vi "nanocal -- nuclear schottky goodness V4.vi"(6 "parameters IN":map{T1, dbl}(c390), 7 "weighting strategy":T2, 8 "dz/dω IN (V)":cdb[](array[numeric])=[1.7183506006211996e-05+0.0i, 1.7124360968751133e-05+0.0i, 1.7049104347380084e-05+0.0i, 1.700437896335042e-05+0.0i, 1.6984579723285106e-05+0.0i, 1.702277369054923e-05+0.0i, 1.713094025845651e-05+0.0i, 1.734249707866828e-05+0.0i, 1.768320429215342e-05+0.0i, 1.8195281152538477e-05+0.0i, 1.8917228661806973e-05+0.0i, 1.9897834564883332e-05+0.0i, 2.154104046962704e-05+0.0i, 2.3247799321765792e-05+0.0i, 2.5364678450551808e-05+0.0i, 2.8645788781885885e-05+0.0i, 3.204749554800641e-05+0.0i, 3.783559691555022e-05+0.0i, 4.245015867332296e-05+0.0i, 4.909131821431355e-05+0.0i, 5.511821898441184e-05+0.0i, 6.178843506022867e-05+0.0i, 7.1079604965352e-05+0.0i, 7.922304381453334e-05+0.0i, 8.814778883893872e-05+0.0i, 9.806709148886077e-05+0.0i, 0.00011119043245647465+0.0i, 0.00012253184919712196+0.0i, 0.00013777724317049346+0.0i, 0.0001508081004573332+0.0i, 0.00016547294918783876+0.0i, 0.00018003847596605868+0.0i, 0.00019518361086534857+0.0i, 0.00021134179818259658+0.0i, 0.0002372041782935464+0.0i, 0.00025518143132024254+0.0i, 0.0002835129702467886+0.0i, 0.0003060118087631287+0.0i, 0.00032860772064336976+0.0i, 0.0003492674091322389+0.0i, 0.00037498324855458583+0.0i, 0.00040021078021115026+0.0i, 0.00041969942568205823+0.0i, 0.00044367338947118773+0.0i, 0.0004634793607238068+0.0i, 0.00047921028781215815+0.0i, 0.0004880906353641744+0.0i, 0.0004932212623741357+0.0i, 0.000491476456593048+0.0i, 0.000480893803992059+0.0i, 0.0004535995818650303+0.0i, 0.000417087772881063+0.0i, 0.0003564148692854789+0.0i, 0.0003049201646356487+0.0i, 0.00021260191240459413+0.0i, 0.00011714858948470126+0.0i, 1.675457544365132e-05+0.0i, -6.8674075405897e-05+0.0i, -0.000156473047607305+0.0i, -0.00026709373934749337+0.0i, -0.0003544271565676041+0.0i, -0.00047937600197311275+0.0i, -0.0006086290582260493+0.0i, -0.0007031877411848573+0.0i, -0.0007564526901441745+0.0i, -0.000802489180995596+0.0i, -0.0008414596018105983+0.0i, -0.0008809346482248761+0.0i, -0.0009073902840241921+0.0i, -0.0009264953054508651+0.0i, -0.0009405659412141811+0.0i, -0.000951649722530156+0.0i, -0.0009557485581057351+0.0i, -0.0009558464741053665+0.0i, -0.0009509110176922098+0.0i, -0.0009411315169847015+0.0i, -0.0009303400913929496+0.0i, -0.0009171113529290538+0.0i, -0.0009022111527275027+0.0i, -0.0008813746494947608+0.0i, -0.0008581837971946129+0.0i, -0.0008372063466683705+0.0i, -0.0008165626610594428+0.0i, -0.0007901155435838691+0.0i, -0.0007682834352800848+0.0i, -0.000746231015527196+0.0i, -0.0007238798463130141+0.0i, -0.0007015567569177018+0.0i, -0.000679301954671598+0.0i, -0.0006572001413831251+0.0i, -0.000629855254567978+0.0i, -0.0006083942229188815+0.0i, -0.0005768631156754208+0.0i, -0.0005562177438951648+0.0i, -0.0005359092039599222+0.0i, -0.0005145186443378148+0.0i, -0.0004951602053444319+0.0i, -0.00047624970229075174+0.0i, -0.0004577401041527736+0.0i, -0.00043519037796120065+0.0i], 9 "Voltage IN (V)":cdb[](array[numeric])=[1.7183506006211996e-05+0.0i, 1.7124360968751133e-05+0.0i, 1.7049104347380084e-05+0.0i, 1.700437896335042e-05+0.0i, 1.6984579723285106e-05+0.0i, 1.702277369054923e-05+0.0i, 1.713094025845651e-05+0.0i, 1.734249707866828e-05+0.0i, 1.768320429215342e-05+0.0i, 1.8195281152538477e-05+0.0i, 1.8917228661806973e-05+0.0i, 1.9897834564883332e-05+0.0i, 2.154104046962704e-05+0.0i, 2.3247799321765792e-05+0.0i, 2.5364678450551808e-05+0.0i, 2.8645788781885885e-05+0.0i, 3.204749554800641e-05+0.0i, 3.783559691555022e-05+0.0i, 4.245015867332296e-05+0.0i, 4.909131821431355e-05+0.0i, 5.511821898441184e-05+0.0i, 6.178843506022867e-05+0.0i, 7.1079604965352e-05+0.0i, 7.922304381453334e-05+0.0i, 8.814778883893872e-05+0.0i, 9.806709148886077e-05+0.0i, 0.00011119043245647465+0.0i, 0.00012253184919712196+0.0i, 0.00013777724317049346+0.0i, 0.0001508081004573332+0.0i, 0.00016547294918783876+0.0i, 0.00018003847596605868+0.0i, 0.00019518361086534857+0.0i, 0.00021134179818259658+0.0i, 0.0002372041782935464+0.0i, 0.00025518143132024254+0.0i, 0.0002835129702467886+0.0i, 0.0003060118087631287+0.0i, 0.00032860772064336976+0.0i, 0.0003492674091322389+0.0i, 0.00037498324855458583+0.0i, 0.00040021078021115026+0.0i, 0.00041969942568205823+0.0i, 0.00044367338947118773+0.0i, 0.0004634793607238068+0.0i, 0.00047921028781215815+0.0i, 0.0004880906353641744+0.0i, 0.0004932212623741357+0.0i, 0.000491476456593048+0.0i, 0.000480893803992059+0.0i, 0.0004535995818650303+0.0i, 0.000417087772881063+0.0i, 0.0003564148692854789+0.0i, 0.0003049201646356487+0.0i, 0.00021260191240459413+0.0i, 0.00011714858948470126+0.0i, 1.675457544365132e-05+0.0i, -6.8674075405897e-05+0.0i, -0.000156473047607305+0.0i, -0.00026709373934749337+0.0i, -0.0003544271565676041+0.0i, -0.00047937600197311275+0.0i, -0.0006086290582260493+0.0i, -0.0007031877411848573+0.0i, -0.0007564526901441745+0.0i, -0.000802489180995596+0.0i, -0.0008414596018105983+0.0i, -0.0008809346482248761+0.0i, -0.0009073902840241921+0.0i, -0.0009264953054508651+0.0i, -0.0009405659412141811+0.0i, -0.000951649722530156+0.0i, -0.0009557485581057351+0.0i, -0.0009558464741053665+0.0i, -0.0009509110176922098+0.0i, -0.0009411315169847015+0.0i, -0.0009303400913929496+0.0i, -0.0009171113529290538+0.0i, -0.0009022111527275027+0.0i, -0.0008813746494947608+0.0i, -0.0008581837971946129+0.0i, -0.0008372063466683705+0.0i, -0.0008165626610594428+0.0i, -0.0007901155435838691+0.0i, -0.0007682834352800848+0.0i, -0.000746231015527196+0.0i, -0.0007238798463130141+0.0i, -0.0007015567569177018+0.0i, -0.000679301954671598+0.0i, -0.0006572001413831251+0.0i, -0.000629855254567978+0.0i, -0.0006083942229188815+0.0i, -0.0005768631156754208+0.0i, -0.0005562177438951648+0.0i, -0.0005359092039599222+0.0i, -0.0005145186443378148+0.0i, -0.0004951602053444319+0.0i, -0.00047624970229075174+0.0i, -0.0004577401041527736+0.0i, -0.00043519037796120065+0.0i], 10 "ω (rad/sec)":dbl[](array[numeric])=[32012.991918577427, 32390.261658505893, 32466.39798177853, 32499.14340521798, 32517.39286113775, 32529.046092051318, 32537.14525712326, 32543.111142615544, 32547.696343954158, 32551.33675949651, 32554.302325209504, 32556.769142360055, 32558.856995237307, 32560.650202739795, 32562.209843476354, 32563.58125099723, 32564.7987833122, 32565.88895894197, 32566.872575330308, 32567.766175404246, 32568.583086316496, 32569.334166794306, 32570.02835688638, 32570.673085530187, 32571.274580490695, 32571.838104118455, 32572.36813539066, 32572.868514009202, 32573.342552524307, 32573.793126289274, 32574.222746575288, 32574.633618125405, 32575.027687968828, 32575.40668442971, 32575.772149741057, 32576.12546690325, 32576.467883345118, 32576.800529469096, 32577.124435064776, 32577.440543590797, 32577.749724325146, 32578.052781957467, 32578.35046682089, 32578.643482565894, 32578.932492128843, 32579.218126471686, 32579.500987779396, 32579.781656707495, 32580.06069600583, 32580.338656060805, 32580.616078519142, 32580.89350097748, 32581.171461032456, 32581.45050033079, 32581.73116925889, 32582.0140305666, 32582.29966469628, 32582.58867447239, 32582.88169000423, 32583.179375080817, 32583.48243271314, 32583.791613234323, 32584.10772197351, 32584.43162756919, 32584.764273480003, 32585.106690135035, 32585.460007297228, 32585.825472395412, 32586.204468856296, 32586.59853891288, 32587.009410462997, 32587.439030535847, 32587.889604513977, 32588.363642815923, 32588.86402143446, 32589.39405291983, 32589.957576334426, 32590.559071508098, 32591.203800151903, 32591.897990030815, 32592.64907072179, 32593.46598163404, 32594.359581707977, 32595.343197883154, 32596.433373726086, 32597.650906041054, 32599.022313348767, 32600.58195429849, 32602.375161800977, 32604.46301467823, 32606.929831615616, 32609.895397541775, 32613.535812870963, 32618.12101442274, 32624.086899701866, 32632.186064986967, 32643.839295900536, 32662.088751820305, 32694.834175046595, 32770.97049853239]) -> (0 "R norm":dbl=-1.0, 1 "G":dbl=-1.0, 2 "R(ω) out":cdb[](array[numeric])=[1.7183506006211996e-05+0.0i, 1.7124360968751133e-05+0.0i, 1.7049104347380084e-05+0.0i, 1.700437896335042e-05+0.0i, 1.6984579723285106e-05+0.0i, 1.702277369054923e-05+0.0i, 1.713094025845651e-05+0.0i, 1.734249707866828e-05+0.0i, 1.768320429215342e-05+0.0i, 1.8195281152538477e-05+0.0i, 1.8917228661806973e-05+0.0i, 1.9897834564883332e-05+0.0i, 2.154104046962704e-05+0.0i, 2.3247799321765792e-05+0.0i, 2.5364678450551808e-05+0.0i, 2.8645788781885885e-05+0.0i, 3.204749554800641e-05+0.0i, 3.783559691555022e-05+0.0i, 4.245015867332296e-05+0.0i, 4.909131821431355e-05+0.0i, 5.511821898441184e-05+0.0i, 6.178843506022867e-05+0.0i, 7.1079604965352e-05+0.0i, 7.922304381453334e-05+0.0i, 8.814778883893872e-05+0.0i, 9.806709148886077e-05+0.0i, 0.00011119043245647465+0.0i, 0.00012253184919712196+0.0i, 0.00013777724317049346+0.0i, 0.0001508081004573332+0.0i, 0.00016547294918783876+0.0i, 0.00018003847596605868+0.0i, 0.00019518361086534857+0.0i, 0.00021134179818259658+0.0i, 0.0002372041782935464+0.0i, 0.00025518143132024254+0.0i, 0.0002835129702467886+0.0i, 0.0003060118087631287+0.0i, 0.00032860772064336976+0.0i, 0.0003492674091322389+0.0i, 0.00037498324855458583+0.0i, 0.00040021078021115026+0.0i, 0.00041969942568205823+0.0i, 0.00044367338947118773+0.0i, 0.0004634793607238068+0.0i, 0.00047921028781215815+0.0i, 0.0004880906353641744+0.0i, 0.0004932212623741357+0.0i, 0.000491476456593048+0.0i, 0.000480893803992059+0.0i, 0.0004535995818650303+0.0i, 0.000417087772881063+0.0i, 0.0003564148692854789+0.0i, 0.0003049201646356487+0.0i, 0.00021260191240459413+0.0i, 0.00011714858948470126+0.0i, 1.675457544365132e-05+0.0i, -6.8674075405897e-05+0.0i, -0.000156473047607305+0.0i, -0.00026709373934749337+0.0i, -0.0003544271565676041+0.0i, -0.00047937600197311275+0.0i, -0.0006086290582260493+0.0i, -0.0007031877411848573+0.0i, -0.0007564526901441745+0.0i, -0.000802489180995596+0.0i, -0.0008414596018105983+0.0i, -0.0008809346482248761+0.0i, -0.0009073902840241921+0.0i, -0.0009264953054508651+0.0i, -0.0009405659412141811+0.0i, -0.000951649722530156+0.0i, -0.0009557485581057351+0.0i, -0.0009558464741053665+0.0i, -0.0009509110176922098+0.0i, -0.0009411315169847015+0.0i, -0.0009303400913929496+0.0i, -0.0009171113529290538+0.0i, -0.0009022111527275027+0.0i, -0.0008813746494947608+0.0i, -0.0008581837971946129+0.0i, -0.0008372063466683705+0.0i, -0.0008165626610594428+0.0i, -0.0007901155435838691+0.0i, -0.0007682834352800848+0.0i, -0.000746231015527196+0.0i, -0.0007238798463130141+0.0i, -0.0007015567569177018+0.0i, -0.000679301954671598+0.0i, -0.0006572001413831251+0.0i, -0.000629855254567978+0.0i, -0.0006083942229188815+0.0i, -0.0005768631156754208+0.0i, -0.0005562177438951648+0.0i, -0.0005359092039599222+0.0i, -0.0005145186443378148+0.0i, -0.0004951602053444319+0.0i, -0.00047624970229075174+0.0i, -0.0004577401041527736+0.0i, -0.00043519037796120065+0.0i], 3 "derivatives OUT":map{T1, dbl}(c390))   [LabVIEW 2020]
uses:
  nanocal-goodness-weighting-strategy.ctl
  3-lorentzian-parameters.ctl
  3-lorentzian-heat-response action.ctl
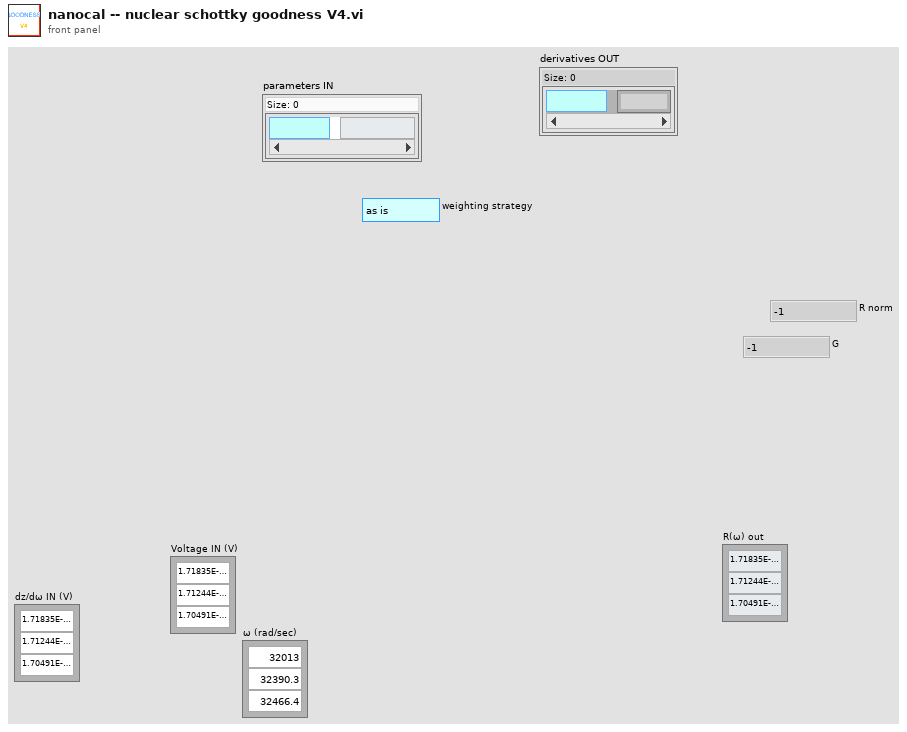
[diagram p1: front panel]
types:
  T1 = typedef "3-lorentzian-parameters.ctl" = enum16{"ζ", "τ1", "τS", "τN", "τC", "κ0", "m1", "m2", "m3", "T (K)", "B (T)", "θ (deg)"}
  T2 = typedef "nanocal-goodness-weighting-strategy.ctl" = enum16{"as is", "|dz/dω|", "ω", "phase"}
  T3 = typedef "3-lorentzian-heat-response action.ctl" = enum16{"calc R", "create string", "calc m1m2m3", "dζ", "dT1", "dτS", "dτN", "dτC", "d-all", "dκ0", "T(K)", "m1", "m2", "m3", "parse string", "θ (deg)", "B (T)", "onlygrads"}
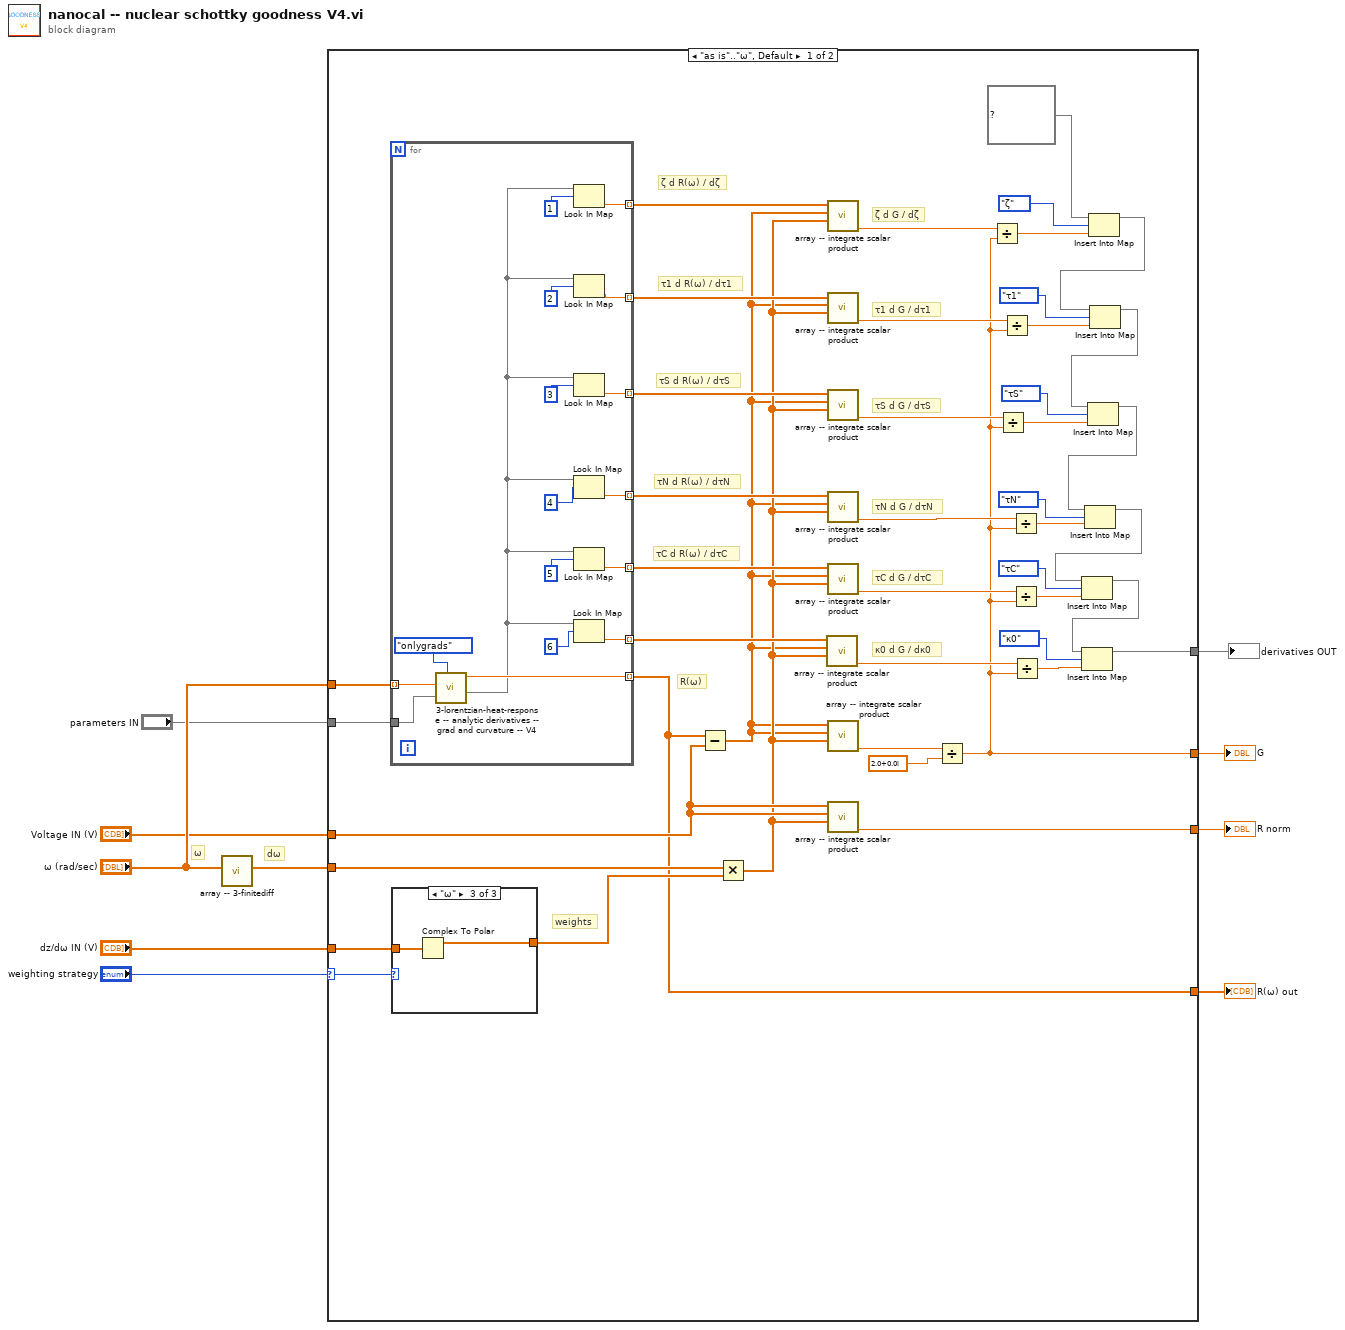
[diagram p0: block diagram]
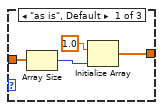
[diagram p2: hidden frame]
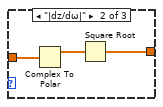
[diagram p3: hidden frame]
diagram:
  # "ω"
  # "dω"
  n1 = call "array -- 3-finitediff.vi"("ω (rad/sec)"="ω (rad/sec)") -> ("dω (rad/sec)"=w10:cdb[])  [unwired: 10 in]
  n2 = case shown="\"as is\"..\"ω\", Default" "weighting strategy" {
    selector: "weighting strategy" -> [w39 _]
    tunnel: w10 -> [w48 _]
    tunnel: "ω (rad/sec)" -> [w47 _]
    tunnel: "Voltage IN (V)" -> [w46 _]
    tunnel: "dz/dω IN (V)" -> [w41 _]
    tunnel: [w30 _] -> w6
    tunnel: [w40 _] -> w5
    tunnel: [w38 _] -> w3
    tunnel: "parameters IN" -> [w37 _]
    tunnel: [w11 _] -> w1
    frame "as is".."ω", Default {
      # "weights"
      # "κ0 d G / dκ0"
      # "τC d G / dτC"
      # "τN d G / dτN"
      # "τS d G / dτS"
      # "τ1 d G / dτ1"
      # "ζ d G / dζ"
      # "τC d R(ω) / dτC"
      # "τN d R(ω) / dτN"
      # "τS d R(ω) / dτS"
      # "τ1 d R(ω) / dτ1"
      # "ζ d R(ω) / dζ"
      # "R(ω)"
      n3 = for {
        tunnel: w47 -> [w79] mode=indexing
        tunnel: [w78] -> w38 mode=indexing
        tunnel: [w76] -> w55 mode=indexing
        tunnel: [w74] -> w54 mode=indexing
        tunnel: [w72] -> w53 mode=indexing
        tunnel: [w70] -> w52 mode=indexing
        tunnel: [w68] -> w51 mode=indexing
        tunnel: [w65] -> w50 mode=indexing
        tunnel: w37 -> [w81]
        n4 = call "3-lorentzian-heat-response -- analytic derivatives -- grad and curvature -- V4.vi"("parameters map  IN"=w81, "action"=3-lorentzian-heat-response_action."onlygrads", "ω (rad/sec)"=w79) -> ("grad map  out"=w66:map{i32, cdb}, "R(ω)"=w78:cdb)  [unwired: 5 in, 2 out]
        n5 = Look In Map(map=w66, key=1 ("index")) -> (value=w76:cdb)  [unwired: 1 in, 1 out]
        n6 = Look In Map(map=w66, key=2 ("index")) -> (value=w74:cdb)  [unwired: 1 in, 1 out]
        n7 = Look In Map(map=w66, key=3 ("index")) -> (value=w72:cdb)  [unwired: 1 in, 1 out]
        n8 = Look In Map(map=w66, key=4 ("index")) -> (value=w70:cdb)  [unwired: 1 in, 1 out]
        n9 = Look In Map(map=w66, key=5 ("index")) -> (value=w68:cdb)  [unwired: 1 in, 1 out]
        n10 = Look In Map(map=w66, key=6 ("index")) -> (value=w65:cdb)  [unwired: 1 in, 1 out]
      }
      n11 = case shown="\"ω\"" w39 {
        tunnel: [w56 w60 w63] -> w43
        tunnel: w41 -> [w58 w62 w64]
        frame "as is", Default {
          n12 = Array Size(array=w58) -> (size(s)=w59:i32)
          n13 = Initialize Array(1.0 ("element"), w59) -> (w56:dbl[])
        }
        frame "|dz/dω|" {
          n14 = Complex To Polar(r * e^(i*theta)=w62) -> (r=w61:dbl[])  [unwired: 1 out]
          n15 = Square Root(x=w61) -> (sqrt(x)=w60:dbl[])
        }
        frame "ω" {
          n16 = Complex To Polar(r * e^(i*theta)=w64) -> (r=w63:dbl[])  [unwired: 1 out]
        }
      }
      n17 = Subtract(x=w38, y=w46) -> (x-y=w42:cdb[])
      n18 = Multiply(x=w48, y=w43) -> (x*y=w45:cdb[])
      n19 = call "array -- integrate scalar product.vi"("dω"=w45, "B"=w42, "A"=w50) -> ("total"=w36:cdb)  [unwired: 7 in, 1 out]
      n20 = call "array -- integrate scalar product.vi"("dω"=w45, "B"=w42, "A"=w55) -> ("total"=w33:cdb)  [unwired: 7 in, 1 out]
      n21 = call "array -- integrate scalar product.vi"("dω"=w45, "B"=w42, "A"=w54) -> ("total"=w31:cdb)  [unwired: 7 in, 1 out]
      n22 = call "array -- integrate scalar product.vi"("dω"=w45, "B"=w42, "A"=w53) -> ("total"=w32:cdb)  [unwired: 7 in, 1 out]
      n23 = call "array -- integrate scalar product.vi"("dω"=w45, "B"=w42, "A"=w52) -> ("total"=w34:cdb)  [unwired: 7 in, 1 out]
      n24 = call "array -- integrate scalar product.vi"("dω"=w45, "B"=w42, "A"=w51) -> ("total"=w35:cdb)  [unwired: 7 in, 1 out]
      n25 = call "array -- integrate scalar product.vi"("dω"=w45, "B"=w42, "A"=w42) -> ("total"=w44:cdb)  [unwired: 7 in, 1 out]
      n26 = call "array -- integrate scalar product.vi"("dω"=w45, "B"=w46, "A"=w46) -> ("total"=w40:cdb)  [unwired: 7 in, 1 out]
      n27 = Divide(x=w44, y=cdb 2.0+0.0i) -> (x/y=w30:cdb)
      n28 = Divide(x=w33, y=w30) -> (x/y=w28:cdb)
      n29 = Divide(x=w32, y=w30) -> (x/y=w24:cdb)
      n30 = Divide(x=w31, y=w30) -> (x/y=w26:cdb)
      n31 = Divide(x=w34, y=w30) -> (x/y=w23:cdb)
      n32 = Divide(x=w35, y=w30) -> (x/y=w20:cdb)
      n33 = Divide(x=w36, y=w30) -> (x/y=w18:cdb)
      n34 = Insert Into Map(map in=map{T1, dbl} {} ("parameters IN"), key=3-lorentzian-parameters."ζ" ("X selector"), value=w28) -> (map out=w27:map{T1, dbl})  [unwired: 2 out]
      n35 = Insert Into Map(map in=w27, key=3-lorentzian-parameters."τ1" ("X selector"), value=w26) -> (map out=w25:map{T1, dbl})  [unwired: 2 out]
      n36 = Insert Into Map(map in=w25, key=3-lorentzian-parameters."τS" ("X selector"), value=w24) -> (map out=w22:map{T1, dbl})  [unwired: 2 out]
      n37 = Insert Into Map(map in=w22, key=3-lorentzian-parameters."τN" ("X selector"), value=w23) -> (map out=w21:map{T1, dbl})  [unwired: 2 out]
      n38 = Insert Into Map(map in=w21, key=3-lorentzian-parameters."τC" ("X selector"), value=w20) -> (map out=w19:map{T1, dbl})  [unwired: 2 out]
      n39 = Insert Into Map(map in=w19, key=3-lorentzian-parameters."κ0" ("X selector"), value=w18) -> (map out=w11:map{T1, dbl})  [unwired: 2 out]
    }
    frame "phase" {
    }
  }
  "G" <- w6
  "R norm" <- w5
  "R(ω) out" <- w3
  "derivatives OUT" <- w1
